vi "Process_IncomingOnly.vi"(8 "error in (no error)":errorcluster, 11 "DebuggingTerminal":refnum<class "DebuggingTerminal.lvclass">) -> ()   [LabVIEW 2013, in "MQTT Base.lvlib"]
uses:
  MQTT Base.lvlib
  DebuggingTerminal.lvclass
  Packet Arrival -- cluster.ctl
  <vilib>/LabVIEW Open Source Project/MQTT Control Packets/Control Packets/ControlPacket/ControlPacket.lvclass
  DebuggingTerminal.lvclass/DebuggingTerminal.ctl
  <vilib>/LabVIEW Open Source Project/MQTT Control Packets/Control Packets/ControlPacket/ControlPacket.lvclass/ControlPacket.ctl
  <vilib>/LabVIEW Open Source Project/MQTT Control Packets/Control Packets/MQTT_311/MQTTVersion.lvclass
  <vilib>/LabVIEW Open Source Project/Advanced Structures/Circular Buffers/VariantBuffer/VariantBuffer.lvclass
  PacketFormatter/PacketFormatter.lvclass
panel:
  in  "auto-scroll IN":bool=TRUE caption="auto-scroll"
  out "Incoming":string
  # "Incoming"
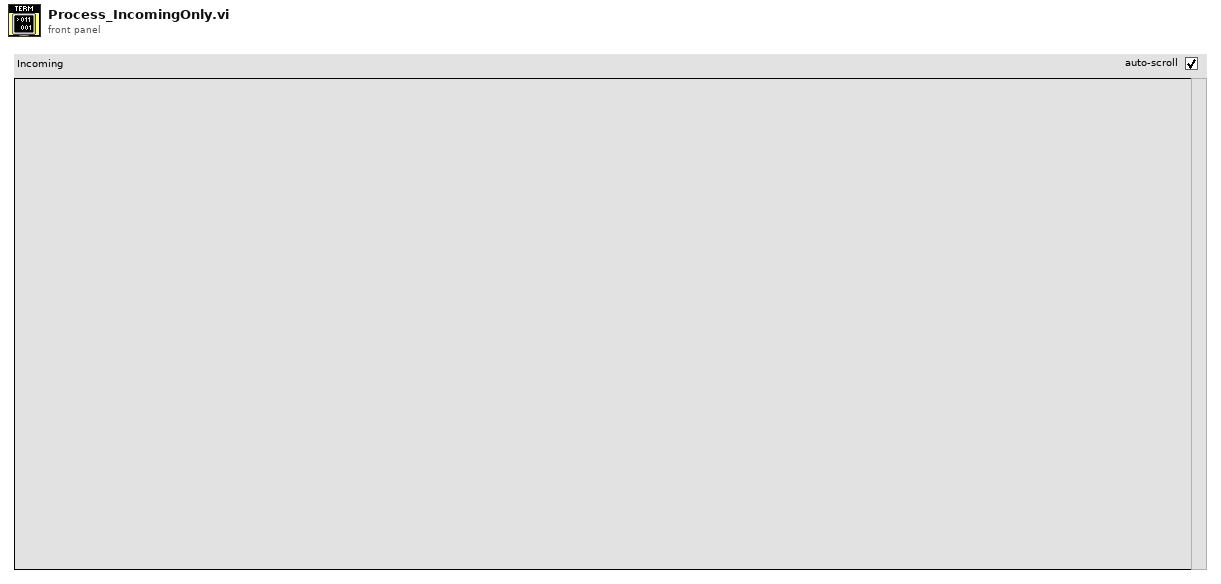
[diagram p1: front panel]
types:
  T1 = typedef "MQTT Base.lvlib/DebuggingTerminal.lvclass/Packet Arrival -- cluster.ctl" = cluster{"Timestamp":timestamp, "Packet":refnum<class "ControlPacket.lvclass">, "Session ID":i32, "outgoing":bool}
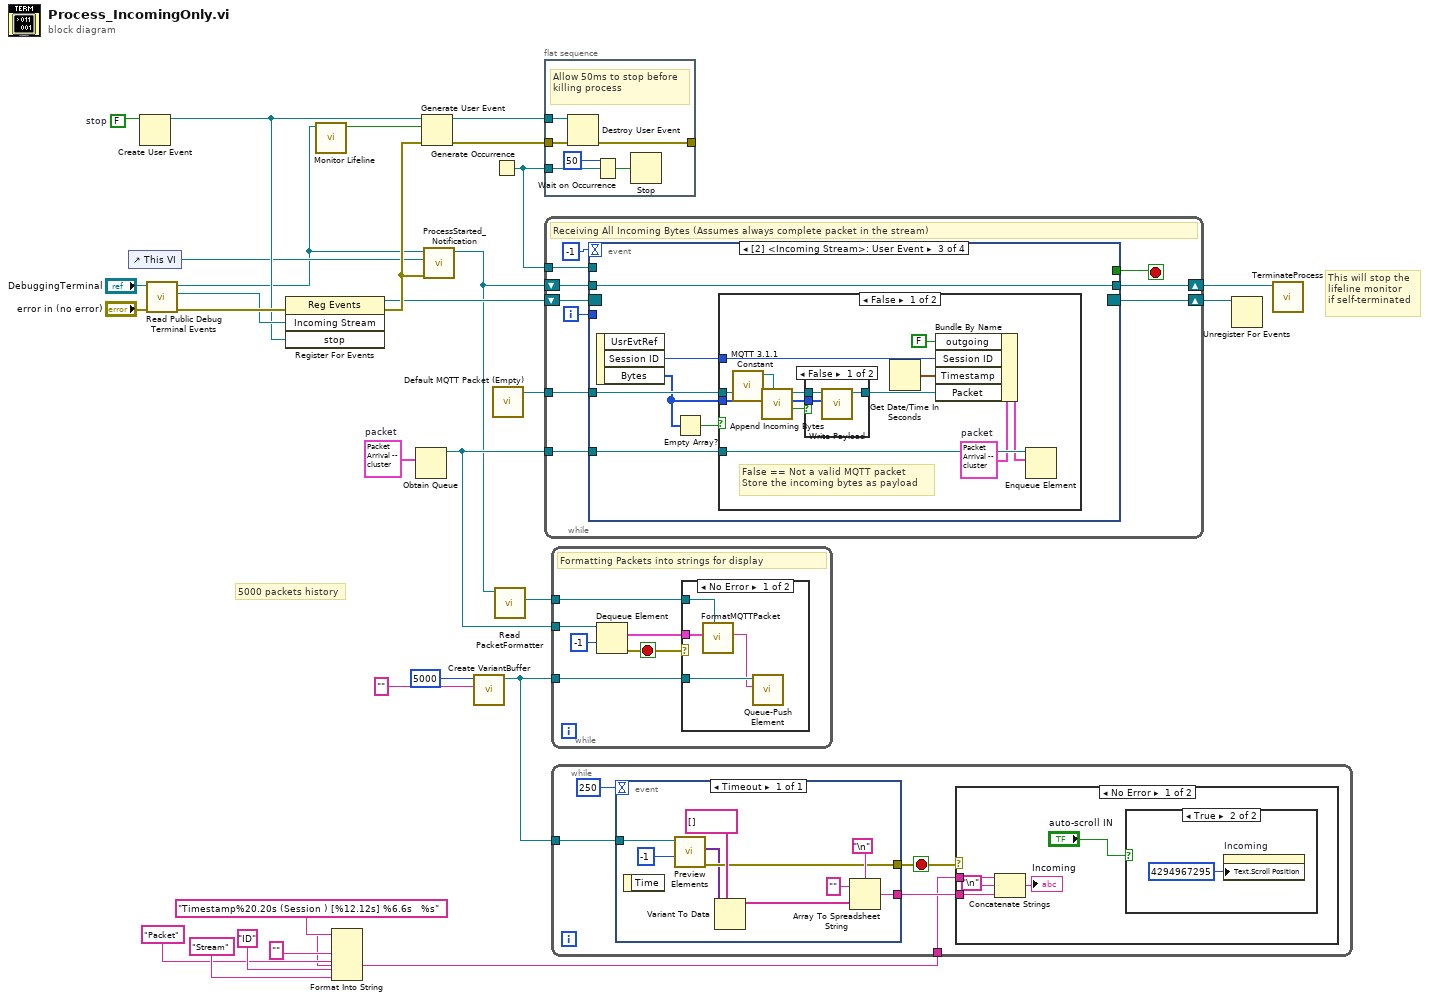
[diagram p0: block diagram]
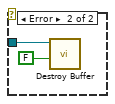
[diagram p4: hidden frame]
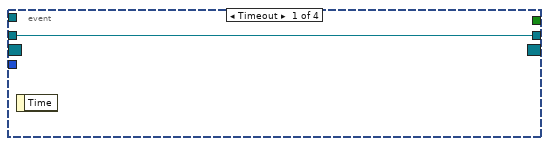
[diagram p5: hidden frame]
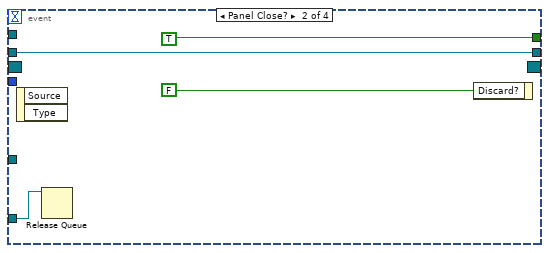
[diagram p6: hidden frame]
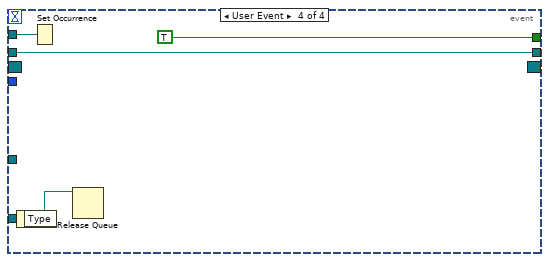
[diagram p9: hidden frame]
diagram:
  w12 = T1 {"Timestamp"=timestamp(0 s since 1904-01-01), "Packet"=refnum, "Session ID"=0, "outgoing"=FALSE}  # packet
  w27 = FALSE  # stop
  # "5000 packets history"
  # "This will stop the\nlifeline monitor\nif self-terminated"
  n1 = control-ref of="This VI"() -> (w11:refnum<vi>)
  n2 = Create User Event(user event datatype=w27) -> (user event=w25:refnum<user-event>)  [unwired: 1 in, 1 out]
  n3 = call "Read Public Debug Terminal Events.vi"("error in (no error)"="error in (no error)", "DebuggingTerminal in"="DebuggingTerminal") -> ("error out"=w29:errorcluster, "Incoming Stream"=w28:refnum<user-event>, "DebuggingTerminal out"=w7:refnum<class "DebuggingTerminal.lvclass">)  [unwired: 6 in, 1 out]
  n4 = register-events(error in=w29, w28, w25) -> (reference out=w4:refnum<event-registration>, error out=w19:errorcluster)  [unwired: 1 in]
  n5 = call "Monitor Lifeline.vi"("DebuggingTerminal in"=w7) -> ("Kill Process"=w26:bool)  [unwired: 10 in]
  n6 = Format Into String(format string="Timestamp%20.20s (Session ) [%12.12s] %6.6s   %s", "" ("input 1"), "Packet" ("input 1"), "ID" ("input 1"), "Stream" ("input 1")) -> (resulting string=w6:string)  [unwired: 2 in, 1 out]
  n7 = Obtain Queue(element data type=w12) -> (queue out=w10:refnum<queue>)  [unwired: 4 in, 2 out]
  n8 = Generate User Event(user event=w25, event data cluster=w26, error in=w19) -> (user event out=w24:refnum<user-event>, error out=w20:errorcluster)  [unwired: 1 in]
  n9 = call "ProcessStarted_Notification.vi"("error in (no error)"=w19, "This VI"=w11, "DebuggingTerminal in"=w7) -> ("DebuggingTerminal out"=w1:refnum<class "DebuggingTerminal.lvclass">)  [unwired: 7 in, 1 out]
  n10 = call <vilib>:"Create VariantBuffer.vi"("default"="" ("input 1"), "bufSize"=5000) -> ("Buffer"=w5:refnum<data-value>)  [unwired: 8 in, 1 out]
  n11 = Generate Occurrence() -> (w23:refnum<k4>)
  n12 = call <vilib>:"Default MQTT Packet (Empty).vi"() -> ("No Packet"=w13:refnum<class "ControlPacket.lvclass">)  [unwired: 11 in]
  n13 = call "Read PacketFormatter.vi"("DebuggingTerminal in"=w1) -> ("PacketFormatter"=w2:refnum<class "PacketFormatter.lvclass">)  [unwired: 9 in, 1 out]
  n14 = flat-sequence {
    tunnel: w24 -> [w36]
    tunnel: w23 -> [w33]
    tunnel: w20 -> [w32]
    tunnel: [w31] -> _
    frame #0 {
      # "Allow 50ms to stop before killing process"
      n15 = Destroy User Event(user event=w36, error in=w32) -> (error out=w31:errorcluster)
      n16 = Wait on Occurrence(2:w33, 3:50 ("ms timeout (-1)")) -> (0:w34:bool)  [unwired: 1 in]
      n17 = Stop(stop? (T)=w34) -> ()
    }
  }
  n18 = while {
    tunnel: w23 -> [w45]
    shift-right: [w43] -> w22
    shift-left: w4 -> [w46]
    shift-right: [w40] -> w21
    shift-left: w1 -> [w41]
    tunnel: w10 -> [w39]
    tunnel: w13 -> [w38]
    i -> [w37]
    stop <- w42 stop-if-true
    # "Receiving All Incoming Bytes (Assumes always complete packet in the stream)"
    n19 = event shown="[2] <Incoming Stream>: User Event" {
      selector: w46 -> [_ _ _ _]
      dyn-events: [_ _ _ _] -> w43
      timeout: -1 -> [_ _ _ _]
      tunnel: w45 -> [_ _ _ w78]
      tunnel: [_ TRUE ("Discard?") _ TRUE] -> w42
      tunnel: w41 -> [w47 w51 w57 w76]
      tunnel: [w47 w51 w57 w76] -> w40
      tunnel: w39 -> [_ w48 w56 w75]
      tunnel: w38 -> [_ _ w54 _]
      tunnel: w37 -> [_ _ _ _]
      event Timeout {
        n20 = event-data() -> ()  [unwired: 1 in, 1 out]
      }
      event Panel Close? {
        n21 = event-data() -> ()  [unwired: 1 in, 2 out]
        n22 = Release Queue(queue=w48) -> ()  [unwired: 2 in, 3 out]
        n23 = event-data("Discard?"=FALSE) -> ()  [unwired: 1 in, 1 out]
      }
      event User Event {
        n24 = event-data() -> ("Session ID"=w55:i32, "Bytes"=w53:u8[])  [unwired: 1 in, 1 out]
        n25 = Empty Array?(array=w53) -> (empty?=w52:bool)
        n26 = case shown="False" w52 {
          tunnel: w56 -> [w69 _]
          tunnel: w55 -> [w68 _]
          tunnel: w54 -> [w67 _]
          tunnel: w53 -> [w59 _]
          frame False {
            w64 = T1 {"Timestamp"=timestamp(0 s since 1904-01-01), "Packet"=refnum, "Session ID"=0, "outgoing"=FALSE}  # packet
            # "False == Not a valid MQTT packet\nStore the incoming bytes as payload"
            n27 = call <vilib>:"MQTT 3.1.1 Constant.vi"() -> ("MQTT 3.1.1"=w70:refnum<class "MQTTVersion.lvclass">)  [unwired: 11 in]
            n28 = call <vilib>:"Append Incoming Bytes.vi"("MQTT Version (3.1.1)"=w70, "Incoming Packets"=w59, "Incomplete ControlPacket"=w67) -> ("Complete Packet"=w63:bool, "Remaining Packets"=w60:u8[], "ControlPacket"=w61:refnum<class "ControlPacket.lvclass">)  [unwired: 5 in, 1 out]
            n29 = case shown="False" w63 {
              tunnel: [w72 w74] -> w62
              tunnel: w61 -> [w73 w74]
              tunnel: w60 -> [w71 _]
              frame False {
                n30 = call <vilib>:"Write Payload.vi"("Payload"=w71, "ControlPacket in"=w73) -> ("ControlPacket out"=w72:refnum<class "ControlPacket.lvclass">)  [unwired: 9 in]
              }
              frame True {
              }
            }
            n31 = Get Date/Time In Seconds() -> (seconds since 1Jan1904=w65:timestamp)
            n32 = Bundle By Name(cluster=w64, "outgoing"=FALSE, "Session ID"=w68, "Timestamp"=w65, "Packet"=w62) -> (w66:T1)
            n33 = Enqueue Element(queue=w69, element=w66) -> ()  [unwired: 2 in, 3 out]
          }
          frame True {
          }
        }
      }
      event User Event {
        n34 = event-data() -> ()  [unwired: 1 in, 1 out]
        n35 = Set Occurrence(w78) -> ()
        n36 = Release Queue(queue=w75) -> ()  [unwired: 2 in, 3 out]
      }
    }
  }
  n37 = while {
    tunnel: w10 -> [w83]
    tunnel: w5 -> [w80]
    tunnel: w2 -> [w79]
    stop <- w84 stop-if-true
    # "Formatting Packets into strings for display"
    n38 = Dequeue Element(queue=w83, timeout in ms (-1)=-1) -> (element=w81:T1, error out=w84:errorcluster)  [unwired: 1 in, 2 out]
    n39 = case shown="No Error" w84 {
      tunnel: w81 -> [w86 _]
      tunnel: w80 -> [w88 w90]
      tunnel: w79 -> [w87 _]
      frame No Error {
        n40 = call "FormatMQTTPacket.vi"("PacketFormatter"=w87, "packet"=w86) -> ("String"=w85:string)  [unwired: 9 in]
        n41 = call <vilib>:"Queue-Push Element.vi"("element"=w85, "Buffer in"=w88) -> ()  [unwired: 5 in, 5 out]
      }
      frame Error {
        n42 = call <vilib>:"Destroy Buffer.vi"("Return Elements (T)"=FALSE, "Buffer"=w90) -> ()  [unwired: 8 in, 2 out]
      }
    }
  }
  n43 = while {
    tunnel: w6 -> [w93]
    tunnel: w5 -> [w91]
    stop <- w92 stop-if-true
    n44 = event shown="[0] Timeout" {
      selector: _ -> [_]
      dyn-events: _ -> [_]
      timeout: 250 -> [_]
      tunnel: [w105] -> w92
      tunnel: [w106] -> w94
      tunnel: w91 -> [w103]
      event Timeout {
        n45 = event-data() -> ()  [unwired: 1 in, 1 out]
        n46 = call <vilib>:"Preview Elements.vi"("count (-1: all)"=-1, "ByteBuffer in"=w103) -> ("error out"=w105:errorcluster, "elements"=w104:variant[])  [unwired: 7 in, 1 out]
        n47 = Variant To Data(type=string[] [], Variant=w104) -> (data=w109:string[])  [unwired: 1 in, 1 out]
        n48 = Array To Spreadsheet String(delimiter (Tab)="\n", array=w109, 3:"" ("format string")) -> (spreadsheet string=w106:string)
      }
    }
    n49 = case shown="No Error" w92 {
      tunnel: w94 -> [w99 _]
      tunnel: w93 -> [w98 _]
      frame No Error {
        n50 = Concatenate Strings(w98, "\n", w99) -> (→"Incoming":string)
        n51 = case shown="True" "auto-scroll IN" {
          frame False {
          }
          frame True {
            n52 = property on="Incoming" class="Str"("Text.Scroll Position"=u32 4294967295) -> ()  [unwired: 2 in, 2 out]
          }
        }
      }
      frame Error {
      }
    }
  }
  n53 = Unregister For Events(event registration refnum=w22) -> ()  [unwired: 1 in, 1 out]
  n54 = call "TerminateProcess.vi"("DebuggingTerminal in"=w21) -> ()  [unwired: 10 in, 1 out]
